vi "Power Accuracy Unflatten Test Parameters.vi"(9 "error in (no error)":errorcluster, 10 "Parameter String":string) -> (1 "error out":errorcluster, 2 "Power Accuracy Test Parameters":T2={"Stimulus"={"Power Start"=38, "Power Stop"=44, "Frequency Type"=enum."Band Edges", "Frequency Points"=[], "TX 1 Frequency (MHz)"={"Min"=0.0, "Max"=0.0}, "TX 2 Frequency (MHz)"={"Min"=0.0, "Max"=0.0}, "RX Frequency (MHz)"={"Min"=0.0, "Max"=0.0}, "Pad Model Number"="", "Pad Serial Number"="", "Pad Values"=[]}, "Measurement"={"DUT Port"=enum."Port 1", "Direction"=0}, "Display"={"Power"={"Min"=0, "Max"=0}, "Tolerance"={"Min"=0.0, "Max"=0.0}}, "Limit"={"Tolerance"=0.35}, "Calibration"={"Calibrated?"=FALSE}} {"Measurement"."Direction" items=["Reverse", "Forward", "Auxiliary"]}, 5 "Test Version":string)   [LabVIEW 2011]
uses:
  TypeDefs/Power Accuracy Test Parameters.ctl
  TypeDefs/Power Accuracy Stimulus Parameters.ctl
  TypeDefs/Power Accuracy Measurement Parameters.ctl
  BPIMCore EXT/HW IO/DUTport.ctl
  BPIMCore EXT/HW IO/MeasMode.ctl
  TypeDefs/Power Accuracy Display Parameters.ctl
  TypeDefs/Power Accuracy Limit Parameters.ctl
  TypeDefs/Power Accuracy Calibration State.ctl
  Test Return Parameter.ctl
panel:
  in  "Return Parameter":T1
  out "Parameter Variant":variant
  in  "Required Instruments":string[](array[string])=["PIM", "PWM"]
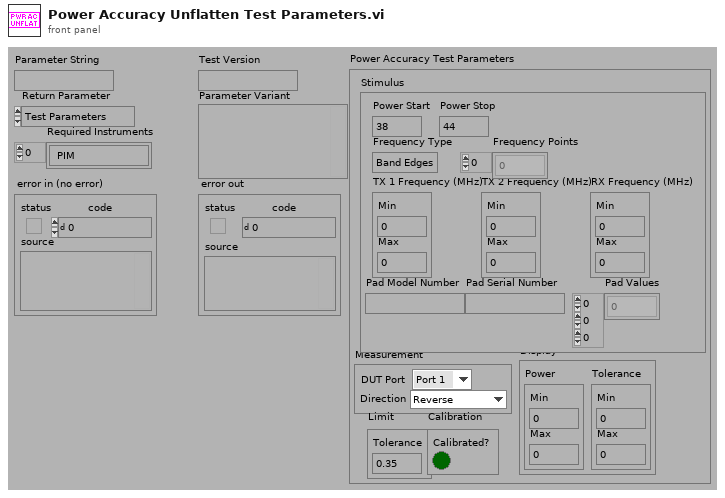
[diagram p1: front panel]
types:
  T1 = typedef "Test Return Parameter.ctl" = enum16{"Test Parameters", "Required Instruments", "Datasheets", "QuickMode"}
  T2 = typedef "Power Accuracy Test Parameters.ctl" = cluster{"Stimulus":T3, "Measurement":T4, "Display":T7, "Limit":T8, "Calibration":T9}
  T3 = typedef "Power Accuracy Stimulus Parameters.ctl" = cluster{"Power Start":i32, "Power Stop":i32, "Frequency Type":enum16{"Band Edges", "Custom"}, "Frequency Points":dbl[], "TX 1 Frequency (MHz)":cluster{"Min":dbl, "Max":dbl}, "TX 2 Frequency (MHz)":cluster{"Min":dbl, "Max":dbl}, "RX Frequency (MHz)":cluster{"Min":dbl, "Max":dbl}, "Pad Model Number":string, "Pad Serial Number":string, "Pad Values":dbl[][][]}
  T4 = typedef "Power Accuracy Measurement Parameters.ctl" = cluster{"DUT Port":T5, "Direction":T6}
  T5 = typedef "DUTport.ctl" = enum16{"Port 1", "Port 2"}
  T6 = typedef "MeasMode.ctl" = u16
  T7 = typedef "Power Accuracy Display Parameters.ctl" = cluster{"Power":cluster{"Min":i32, "Max":i32}, "Tolerance":cluster{"Min":dbl, "Max":dbl}}
  T8 = typedef "Power Accuracy Limit Parameters.ctl" = cluster{"Tolerance":dbl}
  T9 = typedef "Power Accuracy Calibration State.ctl" = cluster{"Calibrated?":bool}
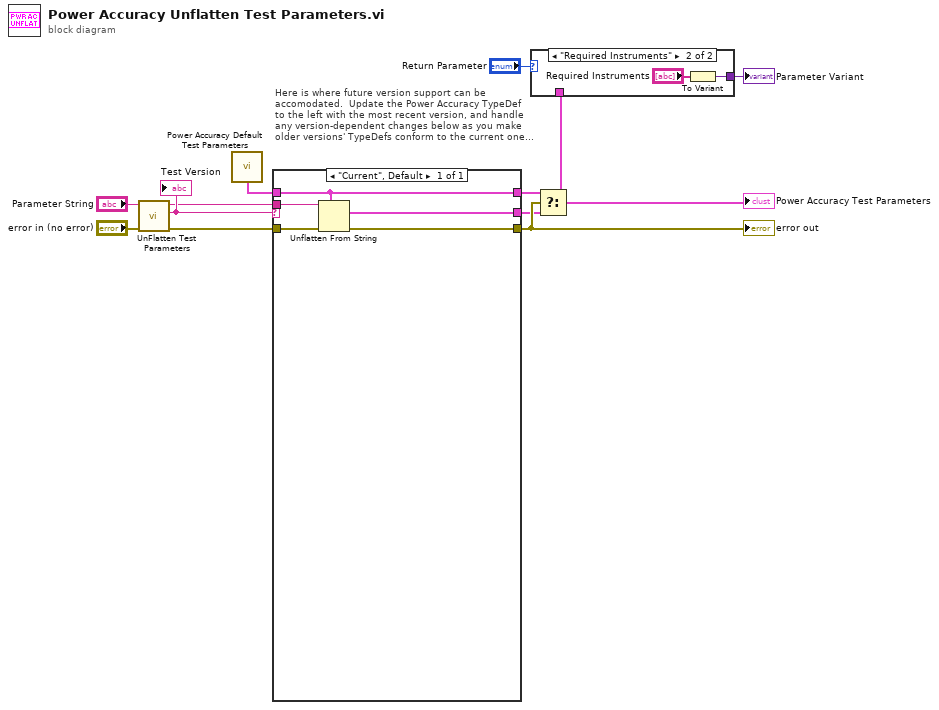
[diagram p0: block diagram]
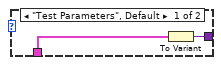
[diagram p2: hidden frame]
diagram:
  # "Here is where future version support can be\naccomodated.  Update the Power Accuracy TypeDef\nto the left with the most recent version, and handle\nany version-dependent changes below as you make\nolder versions' TypeDefs conform to the current one..."
  n1 = call "UnFlatten Test Parameters.vi"("error in (no error)"="error in (no error)", "Flattened Test Parameters with Version (\"\")"="Parameter String") -> ("error out"=w3:errorcluster, "Test Version"=w11:string, "Flat Test Parameters"=w10:string)  [unwired: 3 out]
  "Test Version" <- w11
  n2 = call "Power Accuracy Default Test Parameters.vi"() -> ("Default Power Accuracy Test Parameters"=w1:T2)
  n3 = case shown="\"Current\", Default" w11 {
    tunnel: w10 -> [w17]
    tunnel: w1 -> [w14]
    tunnel: [w16] -> w6
    tunnel: [w14] -> w9
    tunnel: w3 -> [w13]
    tunnel: [w15] -> w2
    frame "Current", Default {
      n4 = Unflatten From String(type=w14, binary string=w17, error in (no error)=w13) -> (value=w15:T2, error out=w16:errorcluster)  [unwired: 3 out]
    }
  }
  "error out" <- w6
  n5 = Select(t=w9, s=w6, f=w2) -> (s? t:f=w5:T2)
  "Power Accuracy Test Parameters" <- w5
  n6 = case shown="\"Required Instruments\"" "Return Parameter" {
    tunnel: [w19 w21] -> w7
    tunnel: w5 -> [w18 _]
    frame "Test Parameters", Default {
      n7 = To Variant(anything=w18) -> (Variant=w19:variant)
    }
    frame "Required Instruments" {
      n8 = To Variant(anything="Required Instruments") -> (Variant=w21:variant)
    }
  }
  "Parameter Variant" <- w7
